vi "DetectExtendCollision.vi"(4 "Ball":T1, 5 "Goal":dbl[](array[numeric]), 6 "Robot in":T2={"id"=0, "function"=enum."Attacker", "x"=0.0, "y"=0.0, "orientation"=0.0, "v_tangent"=0.0, "v_normal"=0.0, "v_ang"=0.0, "kick_x"=0.0, "kick_z"=0.0, "dribble"=FALSE, "Timestamp"=timestamp(0 s since 1904-01-01), "estimatives"={"est_v_tangent"=0.0, "est_v_normal"=0.0, "est_vx"=0.0, "est_vy"=0.0, "Pos Robot Est"=[]}, "dest_x_kick"=0.0, "dest_y_kick"=0.0, "Gap Coord"=[], "States"=enum."GoToTangent", "Path "=[], "Path  Smooth"=[], "Dest"=[]}, 7 "Initial State":dbl[](array[numeric]), 9 "enemy_robots":T2[](array[typedef]), 10 "Point":dbl[](array[numeric]), 11 "our_robots":T2[](array[typedef])) -> (2 "Collision":bool)   [LabVIEW 2018]
uses:
  Core/AI Robot.ctl
  Intel/Functions Enum.ctl
  Intel/AttackerStates.ctl
  PathDests.ctl
  PathDest.ctl
  Core/AI Ball.ctl
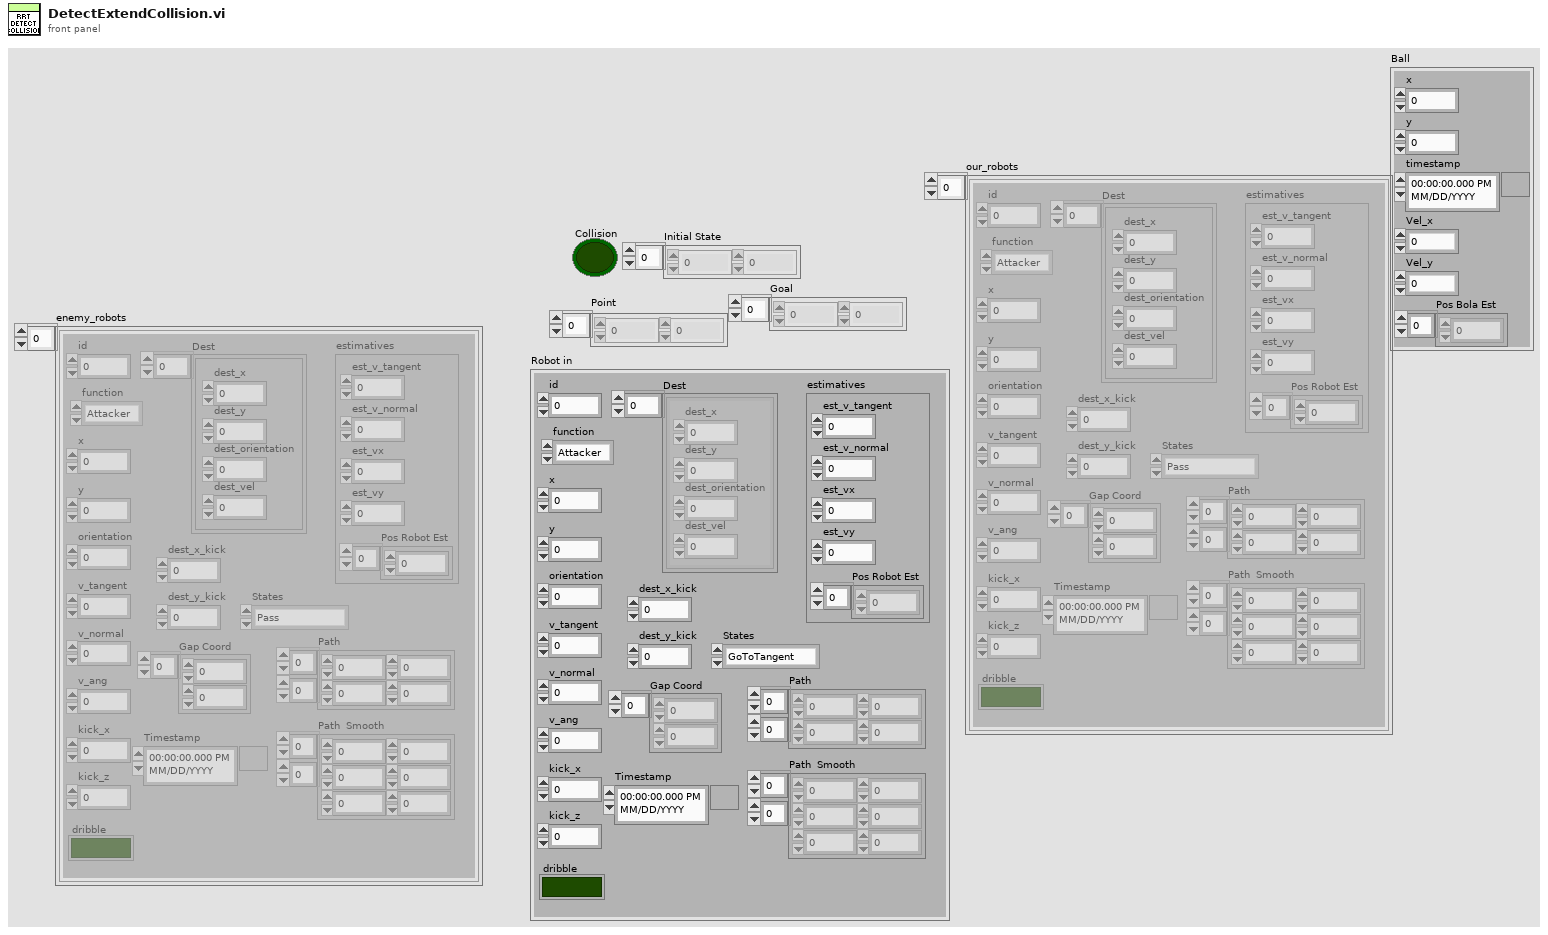
[diagram p1: front panel]
types:
  T1 = typedef "AI Ball.ctl" = cluster{"x":dbl, "y":dbl, "timestamp":timestamp, "Vel_x":dbl, "Vel_y":dbl, "Pos Bola Est":dbl[]}
  T2 = typedef "AI Robot.ctl" = cluster{"id":u32, "function":T3, "x":dbl, "y":dbl, "orientation":dbl, "v_tangent":dbl, "v_normal":dbl, "v_ang":dbl, "kick_x":dbl, "kick_z":dbl, "dribble":bool, "Timestamp":timestamp, "estimatives":cluster{"est_v_tangent":dbl, "est_v_normal":dbl, "est_vx":dbl, "est_vy":dbl, "Pos Robot Est":dbl[]}, "dest_x_kick":dbl, "dest_y_kick":dbl, "Gap Coord":dbl[], "States":T4, "Path ":dbl[][], "Path  Smooth":dbl[][], "Dest":T5}
  T3 = typedef "Functions Enum.ctl" = enum16{"Attacker", "Goalie", "Defender", "Striker", "Goto 0", "Dummy", "Kicker", "ZigZag"}
  T4 = typedef "AttackerStates.ctl" = enum16{"Pass", "GoToTangent", "BallGetting", "GoToKick", "Rotate anti-clockwise", "Rotate Clockwise", ""}
  T5 = typedef "PathDests.ctl" = T6[]
  T6 = typedef "PathDest.ctl" = cluster{"dest_x":dbl, "dest_y":dbl, "dest_orientation":dbl, "dest_vel":dbl}
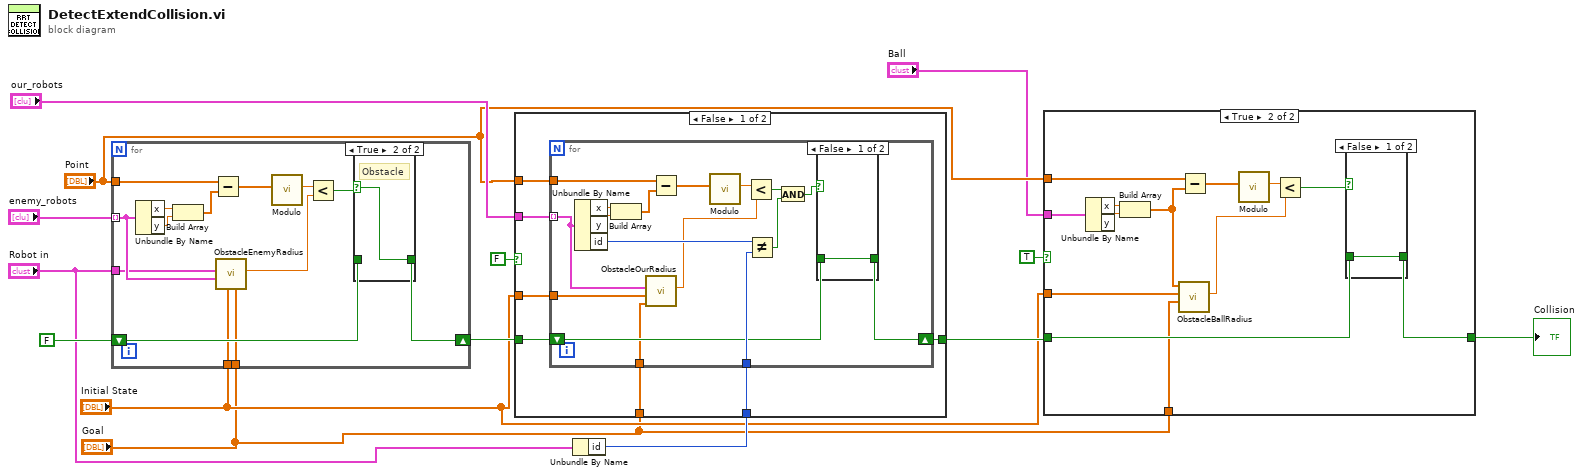
[diagram p0: block diagram]
diagram:
  n1 = for {
    tunnel: "enemy_robots" -> [w18] mode=indexing
    tunnel: "Point" -> [w25]
    shift-right: [w20] -> w9
    shift-left: FALSE -> [w21]
    tunnel: "Robot in" -> [w17]
    tunnel: "Initial State" -> [w16]
    tunnel: "Goal" -> [w15]
    n2 = Unbundle By Name(w18) -> ("x"=w28:dbl, "y"=w27:dbl)
    n3 = Build Array(w28, w27) -> (w26:dbl[])
    n4 = Subtract(x=w25, y=w26) -> (x-y=w24:dbl[])
    n5 = call "ObstacleEnemyRadius.vi"("Goal"=w15, "Initial State"=w16, "Robot enemy"=w18, "Robot in"=w17) -> ("obstacle enemy radius"=w19:dbl)  [unwired: 7 in]
    n6 = call "Modulo.vi"("2D vector"=w24) -> ("Modulo"=w23:dbl)  [unwired: 10 in]
    n7 = Less?(x=w23, y=w19) -> (x < y?=w22:bool)
    n8 = case shown="True" w22 {
      selector: w22 -> [_ w30]
      tunnel: w21 -> [w29 _]
      tunnel: [w29 w30] -> w20
      frame False {
      }
      frame True {
        # "Obstacle"
      }
    }
  }
  n9 = Unbundle By Name("Robot in") -> ("id"=w10:u32)
  n10 = case shown="False" FALSE {
    tunnel: w9 -> [w37 w57]
    tunnel: "our_robots" -> [w36 _]
    tunnel: "Point" -> [w35 _]
    tunnel: [w34 w57] -> w5
    tunnel: w10 -> [w33 _]
    tunnel: "Initial State" -> [w32 _]
    tunnel: "Goal" -> [w31 _]
    frame False {
      n11 = for {
        tunnel: w36 -> [w38] mode=indexing
        tunnel: w35 -> [w51]
        shift-right: [w48] -> w34
        shift-left: w37 -> [w42]
        tunnel: w33 -> [w43]
        tunnel: w32 -> [w40]
        tunnel: w31 -> [w39]
        n12 = Unbundle By Name(w38) -> ("x"=w54:dbl, "y"=w53:dbl, "id"=w44:u32)
        n13 = Build Array(w54, w53) -> (w52:dbl[])
        n14 = call "ObstacleOurRadius.vi"("Goal"=w39, "Initial State"=w40, "other robot"=w38) -> ("obstacle enemy radius"=w41:dbl)  [unwired: 8 in]
        n15 = Subtract(x=w51, y=w52) -> (x-y=w50:dbl[])
        n16 = call "Modulo.vi"("2D vector"=w50) -> ("Modulo"=w49:dbl)  [unwired: 10 in]
        n17 = Less?(x=w49, y=w41) -> (x < y?=w47:bool)
        n18 = Not Equal?(x=w44, y=w43) -> (x != y?=w45:bool)
        n19 = And(x=w47, y=w45) -> (x .and. y?=w46:bool)
        n20 = case shown="False" w46 {
          selector: w46 -> [_ w56]
          tunnel: w42 -> [w55 _]
          tunnel: [w55 w56] -> w48
          frame False {
          }
          frame True {
            # "Obstacle"
          }
        }
      }
    }
    frame True {
    }
  }
  n21 = case shown="True" TRUE {
    tunnel: w5 -> [w58 w71]
    tunnel: "Ball" -> [_ w70]
    tunnel: "Point" -> [_ w69]
    tunnel: [w58 w68] -> w7
    tunnel: "Initial State" -> [_ w61]
    tunnel: "Goal" -> [_ w60]
    frame False {
    }
    frame True {
      n22 = Unbundle By Name(w70) -> ("x"=w64:dbl, "y"=w63:dbl)
      n23 = Build Array(w64, w63) -> (w62:dbl[])
      n24 = call "ObstacleBallRadius.vi"("Goal"=w60, "Initial State"=w61, "ball"=w62) -> ("obstacle enemy radius"=w59:dbl)  [unwired: 8 in]
      n25 = Subtract(x=w69, y=w62) -> (x-y=w67:dbl[])
      n26 = call "Modulo.vi"("2D vector"=w67) -> ("Modulo"=w66:dbl)  [unwired: 10 in]
      n27 = Less?(x=w66, y=w59) -> (x < y?=w65:bool)
      n28 = case shown="False" w65 {
        selector: w65 -> [_ w73]
        tunnel: w71 -> [w72 _]
        tunnel: [w72 w73] -> w68
        frame False {
        }
        frame True {
          # "Obstacle"
        }
      }
    }
  }
  "Collision" <- w7
